vi "Array to Waveform Array.vi"(10 "dt":dbl=1.0, 11 "Array":dbl[](array[numeric])) -> (3 "Waveform":waveform(dbl)[](array[waveform]))   [LabVIEW 2015]
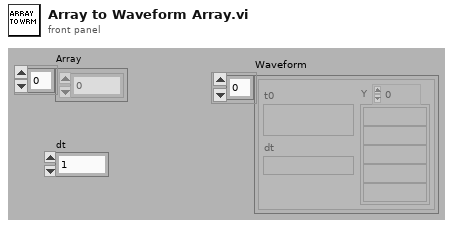
[diagram p1: front panel]
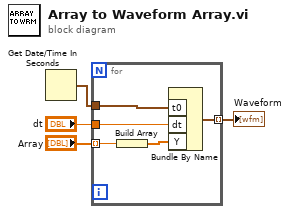
[diagram p0: block diagram]
diagram:
  n1 = Get Date/Time In Seconds() -> (seconds since 1Jan1904=w2:timestamp)
  n2 = for {
    tunnel: "Array" -> [w9] mode=indexing
    tunnel: "dt" -> [w8]
    tunnel: w2 -> [w7]
    tunnel: [w5] -> w1 mode=indexing
    n3 = Build Array(w9) -> (w6:dbl[])
    n4 = Bundle By Name("t0"=w7, "dt"=w8, "Y"=w6) -> (w5:waveform(dbl))  [unwired: 1 in]
  }
  "Waveform" <- w1
